vi "MissionLocation.vi"(8 "error in (no error)":errorcluster, 11 "Idle in":refnum<class "Idle.lvclass">) -> (0 "error out":errorcluster, 2 "bouy location":T1 {"North" format="%#_10f"; "East" format="%#_8f"}, 3 "Idle out":refnum<class "Idle.lvclass">)   [LabVIEW 2013, in "Idle.lvclass"]
uses:
  Idle.lvclass
  Data/TypeDefs/UTM Location.ctl
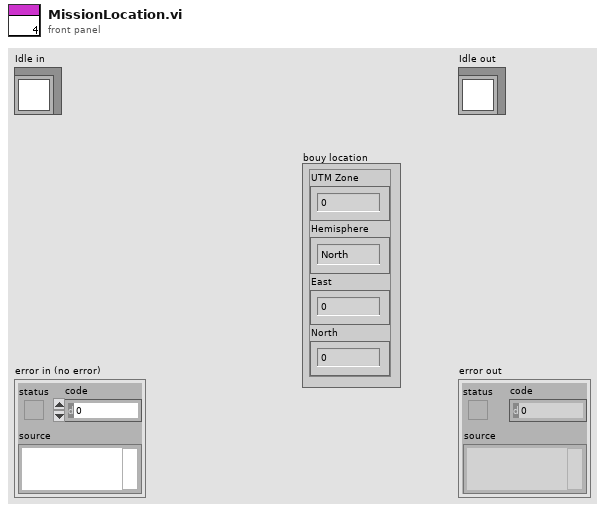
[diagram p1: front panel]
types:
  T1 = typedef "UTM Location.ctl" = cluster{"UTM Zone":dbl, "Hemisphere":enum16{"North", "South"}, "East":dbl, "North":dbl}
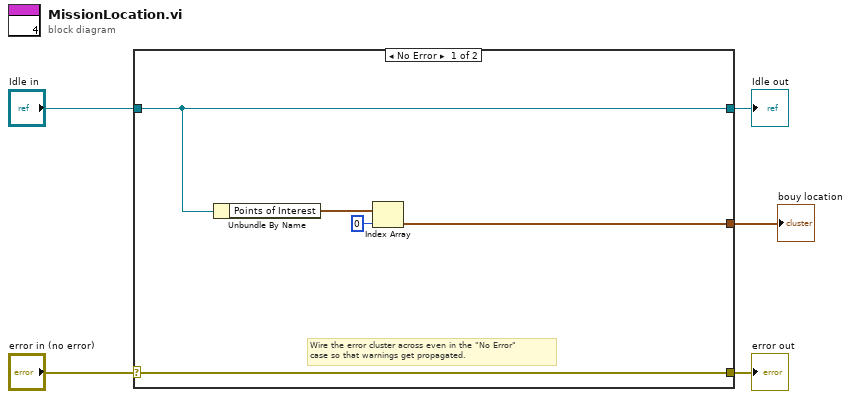
[diagram p0: block diagram]
diagram:
  n1 = case shown="No Error" "error in (no error)" {
    selector: "error in (no error)" -> [w10 w12]
    tunnel: [w10 w12] -> w4
    tunnel: [w7 w11] -> w2
    tunnel: "Idle in" -> [w7 w11]
    tunnel: [w6 _] -> w1
    frame No Error {
      # "Wire the error cluster across even in the \"No Error\"\ncase so that warnings get propagated."
      n2 = Unbundle By Name(w7) -> ("Points of Interest"=w9:T1[])
      n3 = Index Array(array=w9, index=0) -> (element=w6:T1)
    }
    frame Error {
    }
  }
  "error out" <- w4
  "Idle out" <- w2
  "bouy location" <- w1
